vi "Que.-Read.vi"(8 "error in (no error)":errorcluster, 11 "Queue in":refnum<queue>) -> (2 "Boolean":bool, 3 "Output String":string)   [LabVIEW 2016]
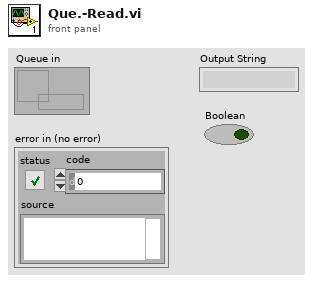
[diagram p1: front panel]
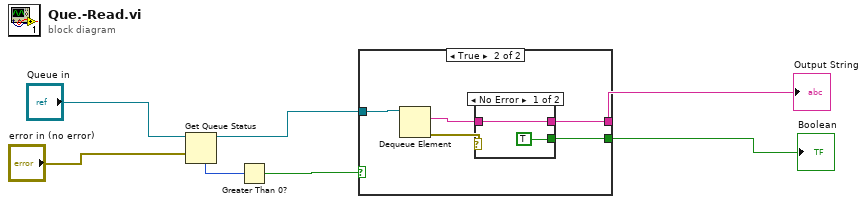
[diagram p0: block diagram]
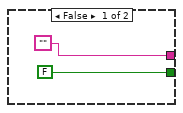
[diagram p2: hidden frame]
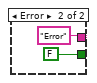
[diagram p3: hidden frame]
diagram:
  n1 = Get Queue Status(queue="Queue in", error in (no error)="error in (no error)") -> (queue out=w1:refnum<queue>, # elements in queue=w2:i32)  [unwired: 1 in, 6 out]
  n2 = Greater Than 0?(x=w2) -> (x > 0?=w3:bool)
  n3 = case shown="True" w3 {
    tunnel: w1 -> [_ w12]
    tunnel: ["" w11] -> w4
    tunnel: [FALSE w10] -> w5
    frame False {
    }
    frame True {
      n4 = Dequeue Element(queue=w12) -> (element=w13:string, error out=w14:errorcluster)  [unwired: 2 in, 2 out]
      n5 = case shown="No Error" w14 {
        tunnel: w13 -> [w16 _]
        tunnel: [w16 "Error"] -> w11
        tunnel: [TRUE FALSE] -> w10
        frame No Error {
        }
        frame Error {
        }
      }
    }
  }
  "Boolean" <- w5
  "Output String" <- w4
